vi "MCP2221_OpenByIndex.vi"(11 "index":u32) -> (0 "error out":errorcluster, 1 "handle out":i32)   [LabVIEW 2025]
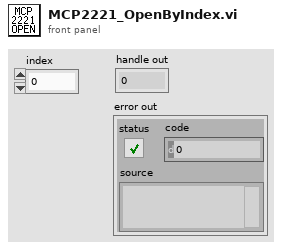
[diagram p1: front panel]
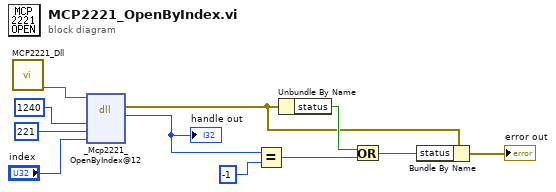
[diagram p0: block diagram]
diagram:
  n1 = call "MCP2221_Dll.vi"() -> ("dll path"=w8:path)  [unwired: 11 in]
  n2 = dll-call lib="?" fn="_Mcp2221_OpenByIndex@12"(path in=w8, "vid"=u32 1240, "pid"=u32 221, "index"="index") -> (error out=w2:errorcluster, "return type"=w7:i32)  [unwired: 5 in, 1 out]
  "handle out" <- w7
  n3 = Equal?(x=w7, y=-1) -> (x = y?=w5:bool)
  n4 = Unbundle By Name(w2) -> ("status"=w6:bool)
  n5 = Or(x=w6, y=w5) -> (x .or. y?=w3:bool)
  n6 = Bundle By Name(cluster=w2, "status"=w3) -> (→"error out":errorcluster)
